vi "Test Abort Parallell Running Tests.vi"(8 "error in (no error)":errorcluster, 11 "Abort Test in":refnum<class "Abort Test.lvclass">) -> (0 "error out":errorcluster, 3 "Abort Test out":refnum<class "Abort Test.lvclass">)   [LabVIEW 2020, in "LUnit Tests.lvlib" / "Abort Test.lvclass"]
uses:
  Abort Test.lvclass
  C:/Program Files (x86)/National Instruments/LabVIEW 2020/vi.lib/Asteme/LUnit/Test Case.lvclass
  source/Framework/Test Suite/LUnit Test Suite.lvclass
  Test Dummys/Hanging Dummy Case/Hanging Dummy Case.lvclass
  C:/Users/anton/Documents/GitHub/LUnit/source/Framework/Test Case/LUnit Test Case.lvclass
  Test Dummys/Hanging Dummy Case 2/Hanging Dummy Case 2.lvclass
  source/Framework/Test Suite/LUnit Test Suite.lvclass/LUnit Test Suite.ctl
  source/Framework/Test Case/LUnit Test Case.lvclass/LUnit Test Case.ctl
  <vilib>/Asteme/LUnit/Test Case.lvclass/Test Case.ctl
  <vilib>/Asteme/LUnit/LUnit Assertion Result.lvclass/LUnit Assertion Result.ctl
  <vilib>/Asteme/LUnit/LUnit Test Case Result.lvclass/LUnit Test Case Result.ctl
  <vilib>/Asteme/LUnit/LUnit Method Result.lvclass/LUnit Method Result.ctl
  source/Framework/Test Case/Public/Accessors/Read Enabled Test Methods.vi
  <vilib>/Asteme/LUnit/Set Assertion Type.vi
  <vilib>/Asteme/LUnit/Palette/Pass.vi
  <vilib>/Asteme/LUnit/Palette/Fail.vi
  <vilib>/Asteme/LUnit/LUnit Write Assertion Type.vi
  <vilib>/Asteme/LUnit/Add test result.vi
  <vilib>/Asteme/LUnit/LUnit Write Passed.vi
  <vilib>/Asteme/LUnit/LUnit Write Message.vi
  <vilib>/Asteme/LUnit/LUnit Write Description.vi
  <vilib>/Asteme/LUnit/LUnit Record Assertion Result.vi
  <vilib>/Asteme/LUnit/LUnit Aggregate Assertion Results.vi
  <vilib>/Asteme/LUnit/Assertion Result/LUnit Read Status.vi
  <vilib>/Asteme/LUnit/LUnit Read Message.vi
  <vilib>/Asteme/LUnit/LUnit Read Description.vi
  <vilib>/Asteme/LUnit/Method Result/LUnit Merge Status.vi
  <vilib>/Asteme/LUnit/LUnit Concatenate result strings.vi
  <vilib>/Asteme/LUnit/LUnit Assertion Result.lvclass
  source/Framework/Execution API/Execution API.lvclass
  <vilib>/Asteme/LUnit/Test Case.lvclass
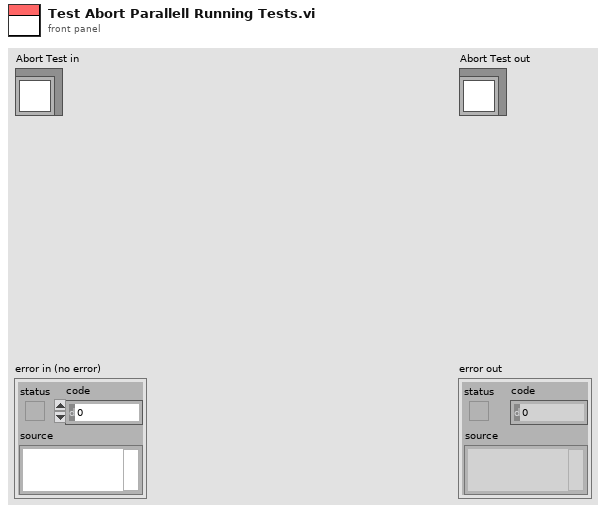
[diagram p1: front panel]
types:
  T1 = cluster{"Event Registration Refnum":refnum<event-registration>, "Event Registration Refnum":refnum<event-registration>}
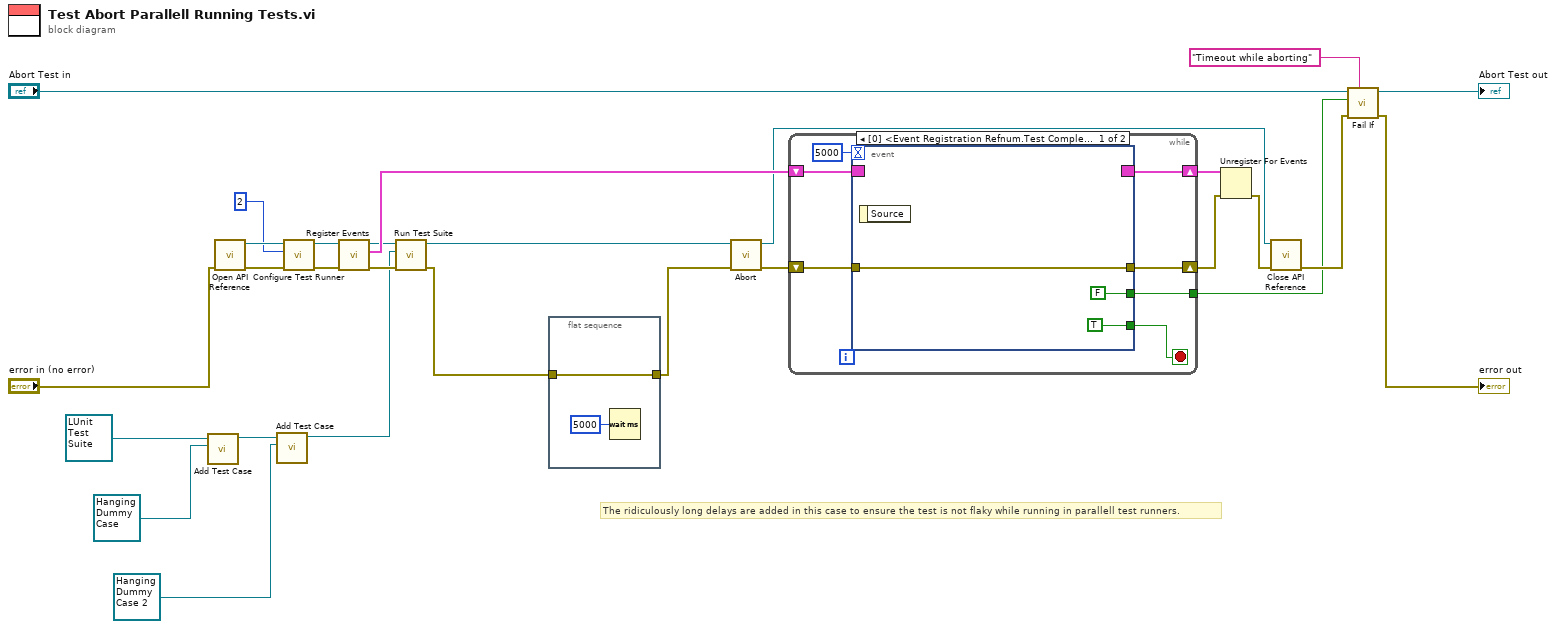
[diagram p0: block diagram]
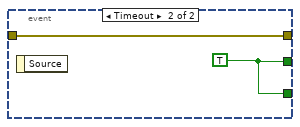
[diagram p2: hidden frame]
diagram:
  # "The ridiculously long delays are added in this case to ensure the test is not flaky while running in parallell test runners."
  n1 = call "Add Test Case.vi"("Test Case to add"=refnum<class "Hanging Dummy Case.lvclass"> refnum ("Hanging Demo Case.lvclass"), "Test Suite In"=refnum<class "LUnit Test Suite.lvclass"> refnum) -> ("Test Suite Out"=w4:refnum<class "LUnit Test Suite.lvclass">)  [unwired: 8 in, 1 out]
  n2 = call "Open API Reference.vi"("error in (no error)"="error in (no error)") -> ("error out"=w11:errorcluster, "Execution API out"=w12:refnum<class "Execution API.lvclass">)  [unwired: 9 in]
  n3 = call "Add Test Case.vi"("Test Case to add"=refnum<class "Hanging Dummy Case 2.lvclass"> refnum ("Hanging Dummy Case 2.lvclass"), "Test Suite In"=w4) -> ("Test Suite Out"=w2:refnum<class "LUnit Test Suite.lvclass">)  [unwired: 8 in, 1 out]
  n4 = call "Configure Test Runner.vi"("error in (no error)"=w11, "Number of Test Runners"=u32 2, "Execution API In"=w12) -> ("error out"=w9:errorcluster, "Execution API Out"=w10:refnum<class "Execution API.lvclass">)  [unwired: 7 in]
  n5 = call "Register Events.vi"("error in (no error)"=w9, "Execution API In"=w10) -> ("error out"=w24:errorcluster, "Result Events"=w25:T1, "Execution API Out"=w23:refnum<class "Execution API.lvclass">)  [unwired: 7 in]
  n6 = call "Run Test Suite.vi"("error in (no error)"=w24, "Test Case"=w2, "Execution API In"=w23) -> ("error out"=w6:errorcluster, "Execution API Out"=w7:refnum<class "Execution API.lvclass">)  [unwired: 7 in]
  n7 = flat-sequence {
    tunnel: [w30] -> w13
    tunnel: w6 -> [w30]
    frame #0 {
      n8 = Wait (ms)(milliseconds to wait=u32 5000) -> ()  [unwired: 1 out]
    }
  }
  n9 = call "Abort.vi"("error in (no error)"=w13, "Execution API in"=w7) -> ("error out"=w14:errorcluster, "Execution API out"=w15:refnum<class "Execution API.lvclass">)  [unwired: 8 in]
  n10 = while {
    shift-right: [w36] -> w26
    shift-left: w25 -> [w37]
    shift-right: [w34] -> w27
    shift-left: w14 -> [w35]
    tunnel: [w32] -> w16
    stop <- w31 stop-if-true
    n11 = event shown="[0] <Event Registration Refnum.Test Completed>: User Event" {
      selector: w37 -> [_ _]
      dyn-events: [_ _] -> w36
      timeout: 5000 -> [_ _]
      tunnel: w35 -> [w40 w42]
      tunnel: [w40 w42] -> w34
      tunnel: [FALSE w41] -> w32
      tunnel: [TRUE w41] -> w31
      event User Event {
        n12 = event-data() -> ()  [unwired: 1 in, 1 out]
      }
      event Timeout {
        w41 = TRUE
        n13 = event-data() -> ()  [unwired: 1 in, 1 out]
      }
    }
  }
  n14 = Unregister For Events(event registration refnum=w26, error in=w27) -> (error out=w28:errorcluster)
  n15 = call "Close API Reference.vi"("error in (no error)"=w28, "Execution API in"=w15) -> ("error out"=w18:errorcluster)  [unwired: 9 in]
  n16 = call <vilib>:"Fail If.vi"("Description"="Timeout while aborting", "error in (no error)"=w18, "Fail?"=w16, "LUnit Test Case In"="Abort Test in") -> ("error out"=→"error out":errorcluster, "LUnit Test Case Out"=→"Abort Test out":refnum<class "Abort Test.lvclass">)  [unwired: 6 in]
